vi "Boost and Slow V.5.0.vi"(11 "Drive Axises":dbl[](array[numeric])) -> ()   [LabVIEW 2016]
uses:
  Robot Global Data V.5.0.vi
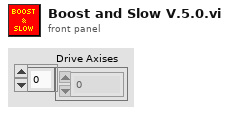
[diagram p1: front panel]
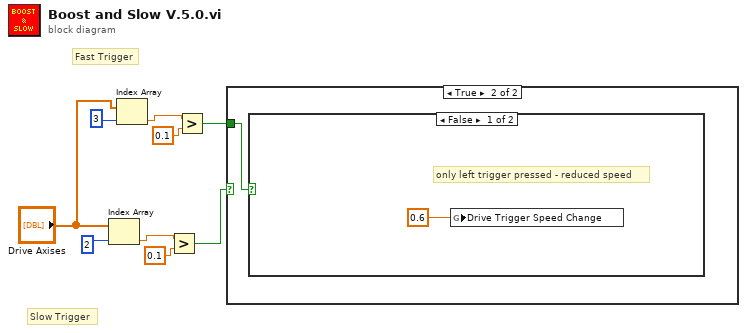
[diagram p0: block diagram]
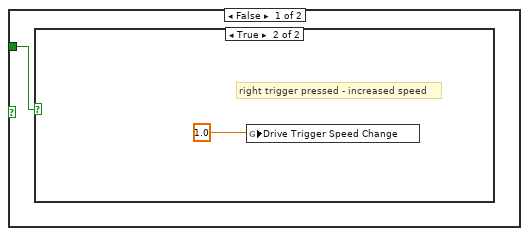
[diagram p2: hidden frame]
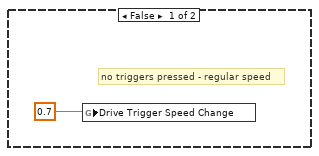
[diagram p3: hidden frame]
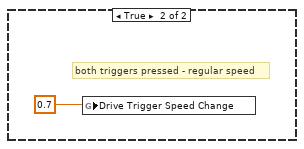
[diagram p4: hidden frame]
diagram:
  # "Fast Trigger"
  # "Slow Trigger"
  n1 = Index Array(array="Drive Axises", index=2) -> (element=w8:dbl)
  n2 = Index Array(array="Drive Axises", index=3) -> (element=w4:dbl)
  n3 = Greater?(x=w8, y=0.1) -> (0:w6:bool)
  n4 = Greater?(x=w4, y=0.1) -> (0:w2:bool)
  n5 = case shown="True" w6 {
    tunnel: w2 -> [w10 w13]
    frame False {
      n6 = case shown="True" w10 {
        frame False {
          # "no triggers pressed - regular speed"
          n7 = global write "Robot Global Data V.5.0.vi" "Drive Trigger Speed Change"(0.7) -> ()
        }
        frame True {
          # "right trigger pressed - increased speed"
          n8 = global write "Robot Global Data V.5.0.vi" "Drive Trigger Speed Change"(1.0) -> ()
        }
      }
    }
    frame True {
      n9 = case shown="False" w13 {
        frame False {
          # "only left trigger pressed - reduced speed"
          n10 = global write "Robot Global Data V.5.0.vi" "Drive Trigger Speed Change"(0.6) -> ()
        }
        frame True {
          # "both triggers pressed - regular speed"
          n11 = global write "Robot Global Data V.5.0.vi" "Drive Trigger Speed Change"(0.7) -> ()
        }
      }
    }
  }
